vi "_FPGA_MSProcess_ParameterHandler.vi"(2 "Init":bool, 3 "Count Increse":bool) -> (0 "Count":u8, 1 "U64 Data":u64)   [LabVIEW 2018]
uses:
  <vilib>/rvi/Emulation/niFpgaEmulationIsFPGAContextNoSignature.vi
  <vilib>/rvi/DataTransferAndStorage/Container/Common/niFpgaContainerGetUniqueNameForEmu.vi
  <vilib>/rvi/Memory/Memory_Emulation/niFpgaMemoryEmulationCacheClearOnFirstRun.vi
  <vilib>/rvi/Memory/Memory_Emulation/nirvimemoryEmulationManagerCache_MakeExclusive.vi
  <vilib>/rvi/Memory/Memory_Emulation/niFpgaMemoryEmulationValidateCache.vi
  <vilib>/rvi/Memory/Memory_Emulation/nirvimemoryEmulationManagerCache_InsertValue.vi
  <vilib>/Utility/error.llb/Clear Errors.vi
  <vilib>/rvi/Memory/Memory_Emulation/nirvimemoryEmulationManagerCache_ReleaseExclusive.vi
  <vilib>/rvi/Memory/Memory_Emulation/nirvimemoryEmulationManagerCache_GetValue.vi
  <vilib>/rvi/Memory/Memory_Emulation/nirvimemoryEmulationManagerCache_SetValue.vi
  <vilib>/rvi/Emulation/niFpgaProcessEmulError.vi
  <vilib>/rvi/Emulation/niFpgaSctlEmulationGetInTimedLoop.vi
  <vilib>/rvi/DataTransferAndStorage/Container/XNode/niFpgaContainer.xnode
  <vilib>/rvi/DataTransferAndStorage/Register/Emulation/niFpgaRegisterEmulation.vi
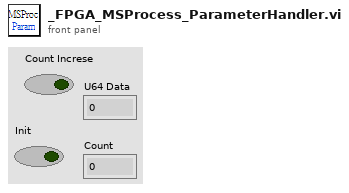
[diagram p1: front panel]
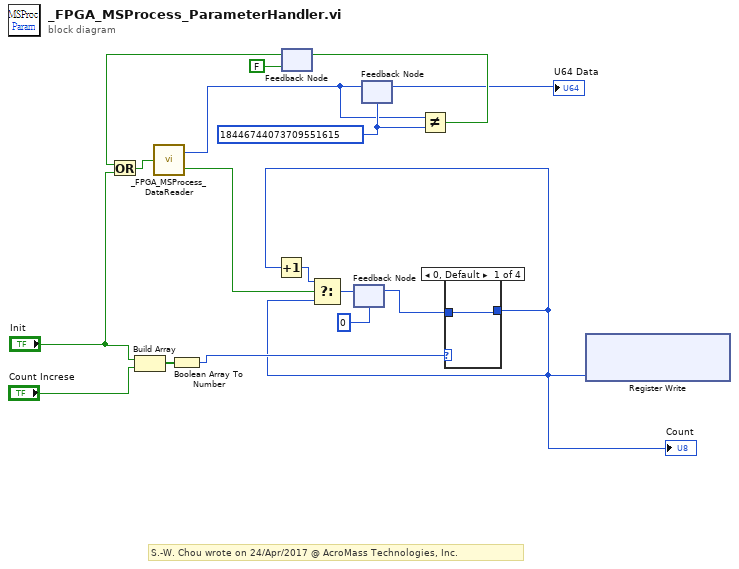
[diagram p0: block diagram]
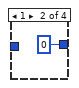
[diagram p2: hidden frame]
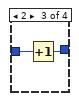
[diagram p3: hidden frame]
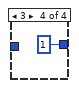
[diagram p4: hidden frame]
diagram:
  w11 = u64 18446744073709551615 ("y")
  # "S.-W. Chou wrote on 24/Apr/2017 @ AcroMass Technologies, Inc."
  n1 = Build Array("Init", "Count Increse") -> (w4:bool[])
  n2 = Boolean Array To Number(Boolean array=w4) -> (number=w3:u8)
  n3 = feedback #1(FALSE) -> (w15:bool)
  n4 = Or(x=w15, y="Init") -> (x .or. y?=w16:bool)
  n5 = call "_FPGA_MSProcess_DataReader.vi"("Read"=w16) -> ("Element"=w9:u64, "new data"=w7:bool)
  n6 = feedback #2(u8 0) -> (w1:u8)
  n7 = feedback-in #3(w9) -> ()
  n8 = feedback #3(w11) -> (→"U64 Data":u64)
  n9 = Not Equal?(x=w9, y=w11) -> (x != y?=w17:bool)
  n10 = feedback-in #1(w17) -> ()
  n11 = case shown="0, Default" w3 {
    tunnel: [w18 u8 0 w20 u8 1] -> w2
    tunnel: w1 -> [w18 _ w21 _]
    frame 0, Default {
    }
    frame 1 {
    }
    frame 2 {
      n12 = Increment(x=w21) -> (x+1=w20:u8)
    }
    frame 3 {
    }
  }
  "Count" <- w2
  n13 = Increment(x=w2) -> (x+1=w14:u8)
  n14 = Select(t=w14, s=w7, f=w2) -> (s? t:f=w12:u8)
  n15 = feedback-in #2(w12) -> ()
  n16 = xnode ("Register Write")("Data"=w2) -> ()  [unwired: 1 in, 1 out]
